vi "TemperatureMonitor.vi"() -> ()   [LabVIEW 2025]
panel:
  out "Temperature History":cluster{dbl, "Thermometer":dbl}(graph)
  in  "Power":bool
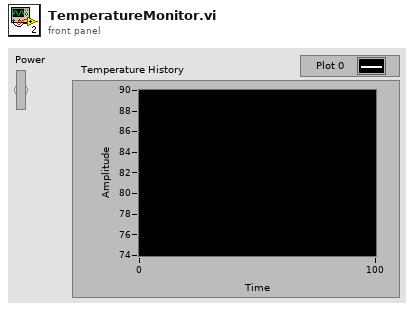
[diagram p1: front panel]
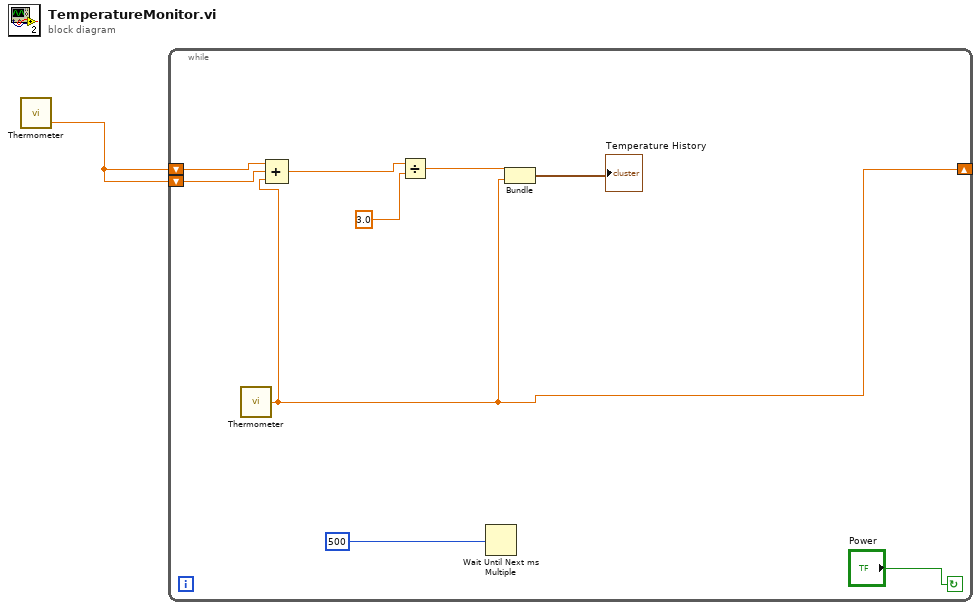
[diagram p0: block diagram]
diagram:
  n1 = call "Thermometer.vi"() -> ("Thermometer"=w1:dbl)  [unwired: 1 in]
  n2 = while {
    shift-right: [w3] -> _
    shift-left: w1 -> [w8]
    shift-left: w1 -> [w7]
    stop <- "Power" continue-if-true
    n3 = call "Thermometer.vi"() -> ("Thermometer"=w3:dbl)  [unwired: 1 in]
    n4 = Compound Arithmetic op=ADD(w8, w7, w3) -> (w6:dbl)
    n5 = Divide(x=w6, y=3.0) -> (x/y=w4:dbl)
    n6 = Wait Until Next ms Multiple(millisecond multiple=500) -> ()  [unwired: 1 out]
    n7 = Bundle(w4, "Thermometer"=w3) -> (→"Temperature History":cluster{dbl, "Thermometer":dbl})  [unwired: 1 in]
  }
